vi "Acquire Data Core.vi"(8 "Error In":errorcluster, 11 "LHW-Aquisition-Actor in":refnum<class "LHW-Aquisition-Actor.lvclass">) -> (0 "Error Out":errorcluster, 2 "LHW-DataCollection":refnum<class "LHW-DataCollection.lvclass">, 3 "LHW-Aquisition-Actor out":refnum<class "LHW-Aquisition-Actor.lvclass">)   [LabVIEW 2014, in "LHW-Acquisition.lvlib" / "LHW-Aquisition-Actor.lvclass"]
doc: "Acquire Data."
uses:
  LHW-Aquisition-Actor.lvclass
  Classes/LHW-Data/LHW-DataCollection/LHW-DataCollection.lvclass
  Classes/LHW-Data/LHW-Data/LHW-Data.lvclass
  Classes/LHW-Data/LHW-Data/LHW-Data.lvclass/LHW-Data.ctl
  Classes/LHW-Data/LHW-DataCollection/LHW-DataCollection.lvclass/LHW-DataCollection.ctl
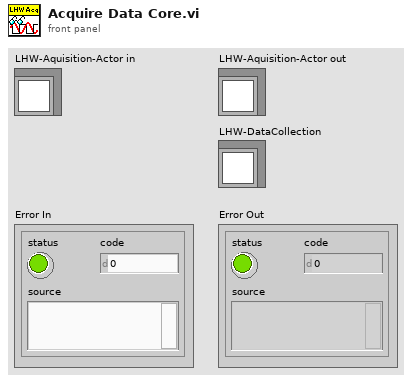
[diagram p1: front panel]
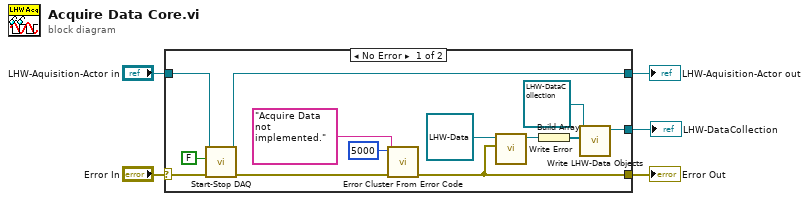
[diagram p0: block diagram]
diagram:
  n1 = case shown="No Error" "Error In" {
    selector: "Error In" -> [w16 w20]
    tunnel: [w10 w20] -> w4
    tunnel: [w12 w19] -> w2
    tunnel: "LHW-Aquisition-Actor in" -> [w13 w19]
    tunnel: [w6 _] -> w1
    frame No Error {
      n2 = call "Start-Stop DAQ.vi"("Error In"=w16, "Start DAQ"=FALSE, "LHW-Aquisition-Actor in"=w13) -> ("Error Out"=w15:errorcluster, "LHW-Aquisition-Actor out"=w12:refnum<class "LHW-Aquisition-Actor.lvclass">)  [unwired: 7 in]
      n3 = call <vilib>:"Error Cluster From Error Code.vi"("error in (no error)"=w15, "error message (\"\")"="Acquire Data not implemented." ("error message (\"\")"), "error code (0)"=5000) -> ("error out"=w10:errorcluster)  [unwired: 6 in]
      n4 = call "Write Error.vi"("Error"=w10, "LHW-Data in"=refnum<class "LHW-Data.lvclass"> refnum ("LHW-Data.lvlib:LHW-Data.lvclass")) -> ("LHW-Data out"=w9:refnum<class "LHW-Data.lvclass">)  [unwired: 8 in, 1 out]
      n5 = Build Array(w9) -> (w7:refnum<class "LHW-Data.lvclass">[])
      n6 = call "Write LHW-Data Objects.vi"("LHW-Data Objects"=w7, "LHW-DataCollection in"=refnum<class "LHW-DataCollection.lvclass"> refnum ("LHW-Data.lvlib:LHW-DataCollection.lvclass")) -> ("LHW-DataCollection out"=w6:refnum<class "LHW-DataCollection.lvclass">)  [unwired: 8 in, 1 out]
    }
    frame Error {
    }
  }
  "Error Out" <- w4
  "LHW-Aquisition-Actor out" <- w2
  "LHW-DataCollection" <- w1
